vi "Get RHS.vi"(8 "error in (no error)":errorcluster, 10 "Domain":refnum<class "NI_Domain.lvclass">, 11 "RHS_3D_Numeric in":refnum<class "NI_RHS_3D_Numeric.lvclass">) -> (0 "error out":errorcluster, 2 "RHS":variant, 3 "RHS_3D_Numeric out":refnum<class "NI_RHS_3D_Numeric.lvclass">)   [LabVIEW 2017, in "NI_PDE.lvlib" / "NI_RHS_3D_Numeric.lvclass"]
uses:
  <vilib>/gmath/pde.llb/RHSClass/RHS_3D_Numeric/NI_RHS_3D_Numeric.lvclass
  <vilib>/gmath/pde.llb/DomainClass/NI_Domain.lvclass
  <vilib>/gmath/pde.llb/RHSClass/RHS_3D_Numeric/NI_RHS_3D_Numeric.lvclass/NI_RHS_3D_Numeric.ctl
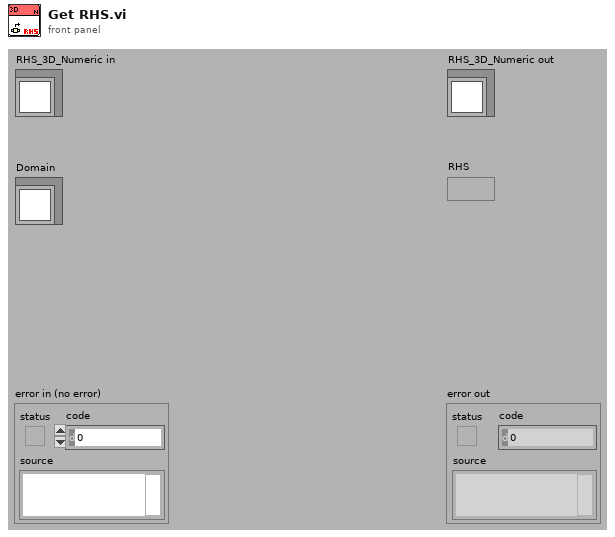
[diagram p1: front panel]
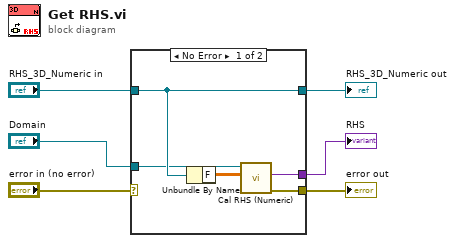
[diagram p0: block diagram]
diagram:
  n1 = case shown="No Error" "error in (no error)" {
    selector: "error in (no error)" -> [_ w12]
    tunnel: "RHS_3D_Numeric in" -> [w11 w13]
    tunnel: [w7 _] -> w5
    tunnel: [w11 w13] -> w4
    tunnel: [w8 w12] -> w3
    tunnel: "Domain" -> [w10 _]
    frame No Error {
      n2 = Unbundle By Name(w11) -> ("F"=w9:dbl[][][])
      n3 = call-dynamic "Cal RHS (Numeric).vi"("RHS in"=w9, "Domain in"=w10) -> ("error out"=w8:errorcluster, "RHS out"=w7:variant)  [unwired: 1 in, 7 out]
    }
    frame Error {
    }
  }
  "RHS" <- w5
  "error out" <- w3
  "RHS_3D_Numeric out" <- w4
